vi "st_Wilcoxon probability lookup.vi"(9 "x":i32, 11 "table column":T1) -> (2 "P{W+ >= x}":dbl)   [LabVIEW 2017, in "NI_Gmath.lvlib"]
uses:
  NI_Gmath.lvlib
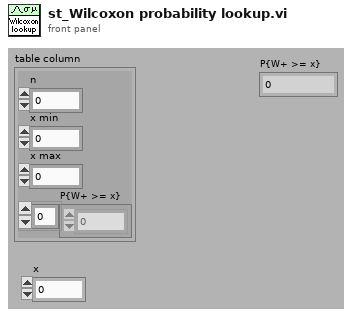
[diagram p1: front panel]
types:
  T1 = cluster{"n":u8, "x min":u8, "x max":u8, "P{W+ >= x}":sgl[]}
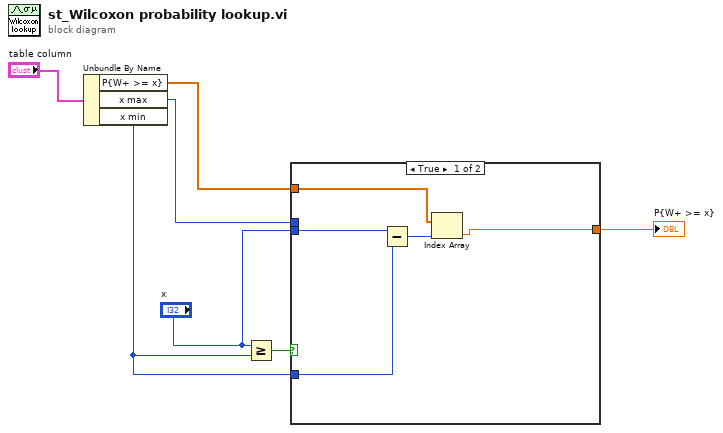
[diagram p0: block diagram]
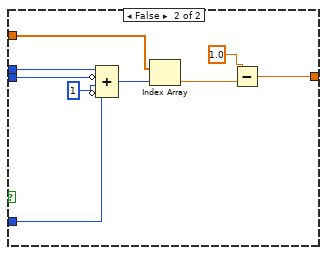
[diagram p2: hidden frame]
diagram:
  n1 = Unbundle By Name("table column") -> ("P{W+ >= x}"=w5:sgl[], "x max"=w3:u8, "x min"=w1:u8)
  n2 = Greater Or Equal?(x="x", y=w1) -> (x >= y?=w6:bool)
  n3 = case shown="True" w6 {
    tunnel: w3 -> [_ w21]
    tunnel: "x" -> [w11 w20]
    tunnel: w5 -> [w12 w17]
    tunnel: [w8 w14] -> w2
    tunnel: w1 -> [w10 w13]
    frame True {
      n4 = Subtract(x=w11, y=w10) -> (x-y=w9:i32)
      n5 = Index Array(array=w12, index=w9) -> (element=w8:sgl)
    }
    frame False {
      n6 = Compound Arithmetic op=ADD(w21, invert w20, 1 ("value"), invert w13) -> (w18:i32)
      n7 = Index Array(array=w17, index=w18) -> (element=w15:sgl)
      n8 = Subtract(x=1.0, y=w15) -> (x-y=w14:dbl)
    }
  }
  "P{W+ >= x}" <- w2
